vi "SetVCLKReg.vi"(1 "vfreq":u8, 2 "lines":u32, 3 "board_sel":u32=1) -> ()   [LabVIEW 2015]
uses:
  ESLSCDLL.dll
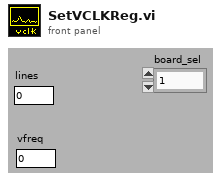
[diagram p1: front panel]
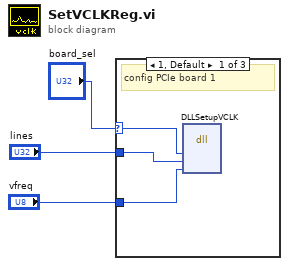
[diagram p0: block diagram]
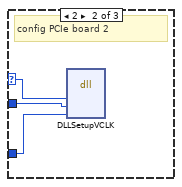
[diagram p2: hidden frame]
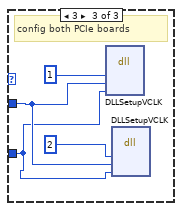
[diagram p3: hidden frame]
diagram:
  n1 = case shown="1, Default" "board_sel" {
    selector: "board_sel" -> [w6 w9 _]
    tunnel: "lines" -> [w5 w8 w11]
    tunnel: "vfreq" -> [w4 w7 w10]
    frame 1, Default {
      # "config PCIe board 1"
      n2 = dll-call lib="C:/ENTW/PCIE/64bit/lv64/board.vis/ESLSCDLL.dll" fn="DLLSetupVCLK"("drv"=w6, "lines"=w5, "vfreq"=w4) -> ()  [unwired: 7 in, 2 out]
    }
    frame 2 {
      # "config PCIe board 2"
      n3 = dll-call lib="C:/ENTW/PCIE/64bit/lv64/board.vis/ESLSCDLL.dll" fn="DLLSetupVCLK"("drv"=w9, "lines"=w8, "vfreq"=w7) -> ()  [unwired: 7 in, 2 out]
    }
    frame 3 {
      # "config both PCIe boards"
      n4 = dll-call lib="C:/ENTW/PCIE/64bit/lv64/board.vis/ESLSCDLL.dll" fn="DLLSetupVCLK"("drv"=u32 1, "lines"=w11, "vfreq"=w10) -> ()  [unwired: 7 in, 2 out]
      n5 = dll-call lib="C:/ENTW/PCIE/64bit/lv64/board.vis/ESLSCDLL.dll" fn="DLLSetupVCLK"("drv"=u32 2, "lines"=w11, "vfreq"=w10) -> ()  [unwired: 7 in, 2 out]
    }
  }
